vi "Test VI.vi"() -> ()   [LabVIEW 2011]
panel:
  in  "Test 1":string
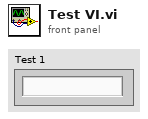
[diagram p1: front panel]
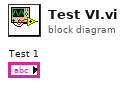
[diagram p0: block diagram]
diagram:
